vi "test19-AsteriskWildcardStateRegistration.vi"(8 "error in (no error)":errorcluster, 11 "TestCase in":refnum<class "testcase-CSMBroadcast.lvclass">) -> (0 "error out":errorcluster, 3 "TestCase out":refnum<class "testcase-CSMBroadcast.lvclass">)   [LabVIEW 2017, in "testcase-CSMBroadcast.lvclass"]
uses:
  testcase-CSMBroadcast.lvclass
  0c20cacf-7d77-4f8e-aec5-f22e7d09936d.vi
  26de337d-8090-412f-9da5-e117a55d4726.vi
  de10340a-d592-45ad-b055-7fa7b377c551.vi
  e3eae2f8-d8ce-4adb-8167-9a417250fce1.vi
  a4d00e00-a9ed-4631-bf53-269bf71f16fc.vi
  src/user.lib/_NEVSTOP/Communicable State Machine(CSM)/AdvanceAPI/CSM - Revert Arguments-Safe String.vi
  src/user.lib/_NEVSTOP/Communicable State Machine(CSM)/AdvanceAPI/CSM - Make String Arguments Safe.vi
  src/user.lib/_NEVSTOP/Communicable State Machine(CSM)/AdvanceAPI/CSM - Break Down Multiple States String.vi
  src/user.lib/_NEVSTOP/Communicable State Machine(CSM)/AdvanceAPI/CSM - Compact Multiple States.vi
  src/user.lib/_NEVSTOP/Communicable State Machine(CSM)/AdvanceAPI/CSM - Keywords.vi
  src/user.lib/_NEVSTOP/Communicable State Machine(CSM)/_Shared/Trim Single-line Text.vi
  src/user.lib/_NEVSTOP/Communicable State Machine(CSM)/AdvanceAPI/CSM - Set Module Attribute.vi
  src/user.lib/_NEVSTOP/Communicable State Machine(CSM)/AdvanceAPI/CSM - Get Module Attribute.vi
  <vilib>/addons/_JKI Toolkits/VI Tester/TestCase.llb/TestCase.lvclass
  src/user.lib/_NEVSTOP/Communicable State Machine(CSM)/Communicable State Machine.lvlib
  CSM/CSM-Testcase.lvlib
  C:/Program Files (x86)/National Instruments/LabVIEW 2017/vi.lib/addons/_JKI Toolkits/VI Tester/TestCase.llb/TestCase.lvclass
panel:
  out "Execution Times":i32
  out "State History":string
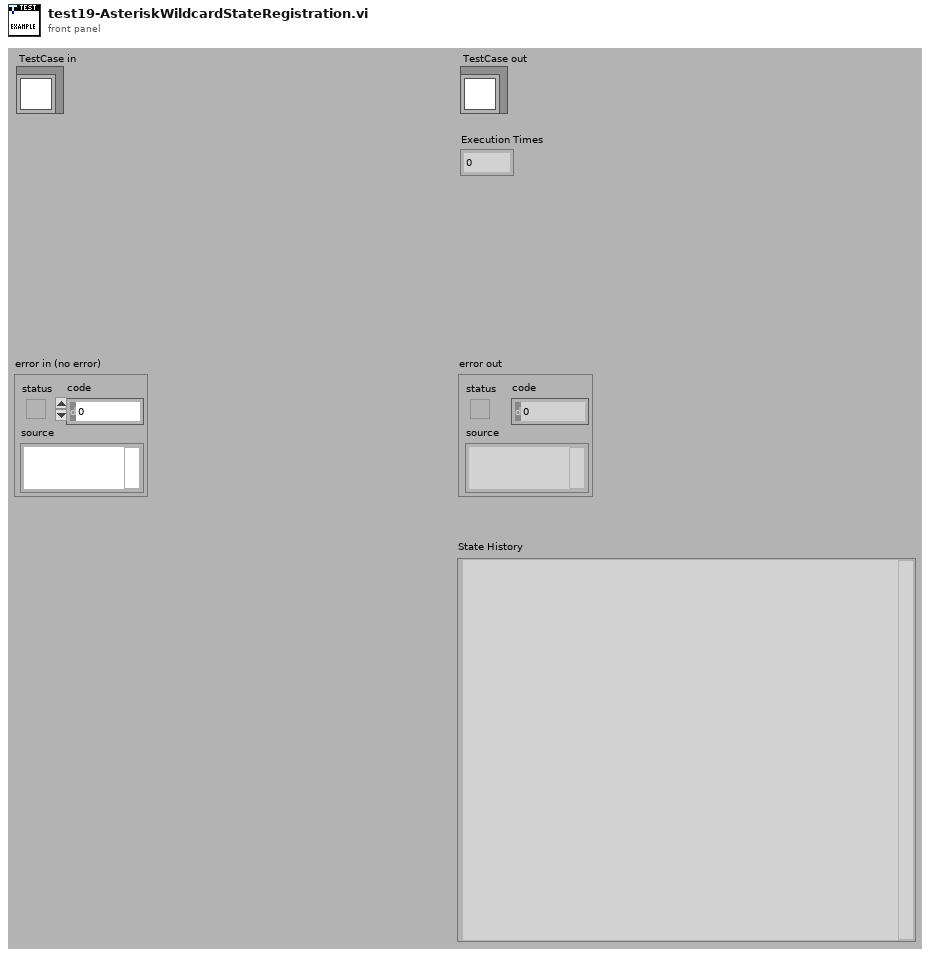
[diagram p1: front panel]
types:
  T1 = enum32{"Invalid", "Standard", "Closed", "Hidden", "Minimized", "Maximized"}
  T2 = enum32{"invalid app kind", "Development System", "Run Time System", "Student Edition", "Embedded LabVIEW", "Evaluation", "Custom"}
  T3 = typedef "Communicable State Machine.lvlib/_CSM_Response Source Message.ctl" = cluster{"‘State":string, "’Arguments":string, "’Error":errorcluster}
  T4 = cluster{"Current VI Reference":refnum<vi>, "Close Panel on Exit?":bool}
  T5 = cluster{"Core":cluster{"Current VI Reference":refnum<vi>, "Close Panel on Exit?":bool}, "Your Boolean data":bool, "Your string data":string, "TestData":i32}
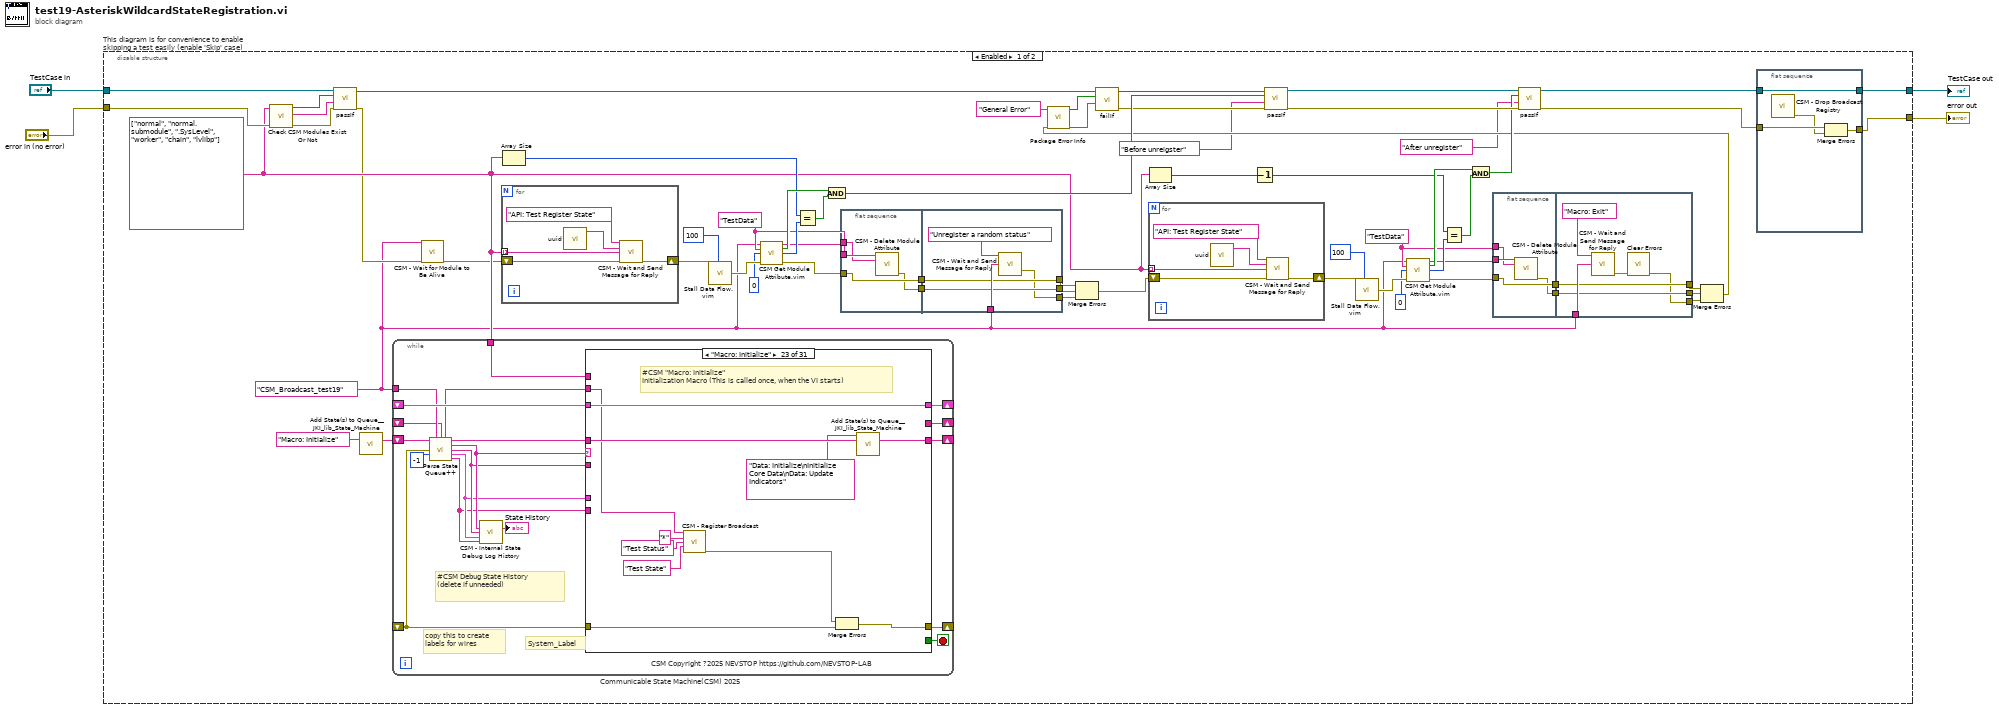
[diagram p0: block diagram]
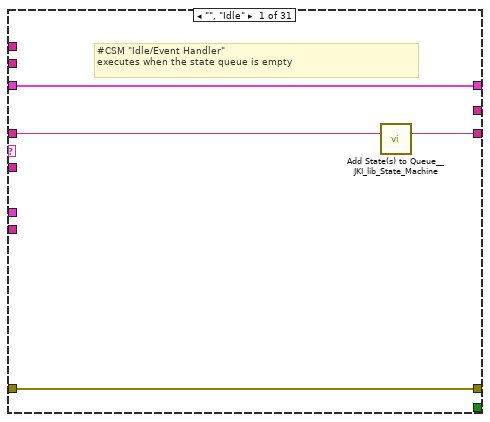
[diagram p2: hidden frame]
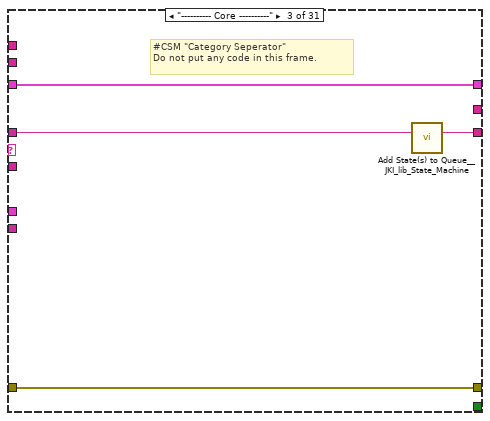
[diagram p4: hidden frame]
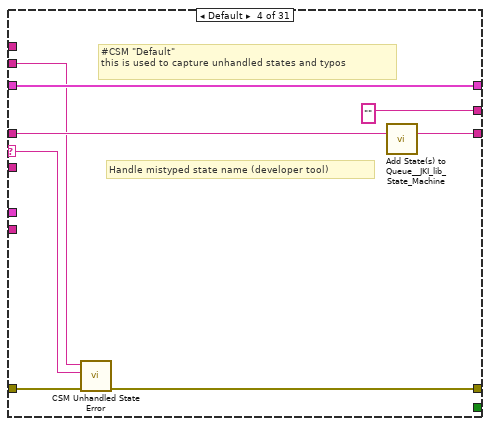
[diagram p5: hidden frame]
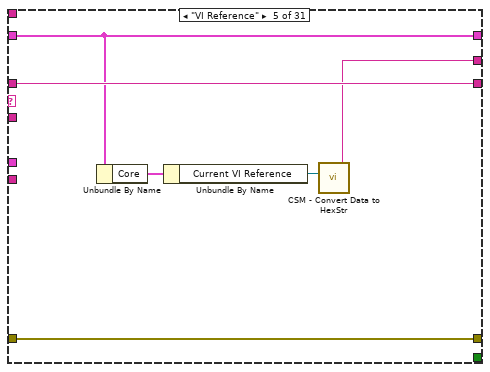
[diagram p6: hidden frame]
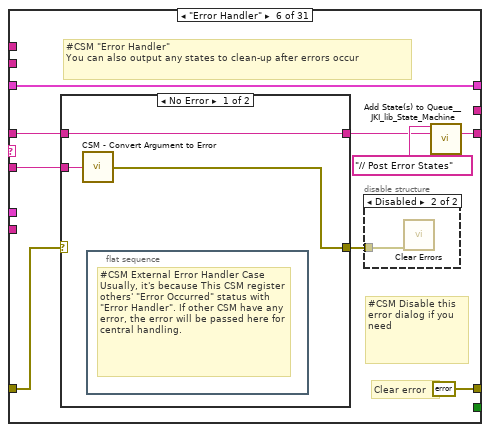
[diagram p7: hidden frame]
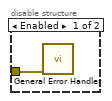
[diagram p8: hidden frame]
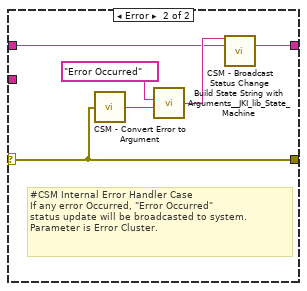
[diagram p9: hidden frame]
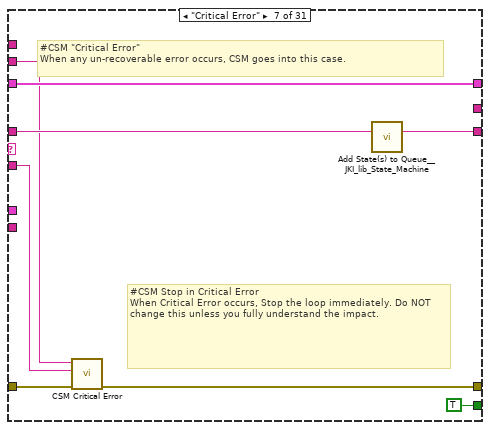
[diagram p10: hidden frame]
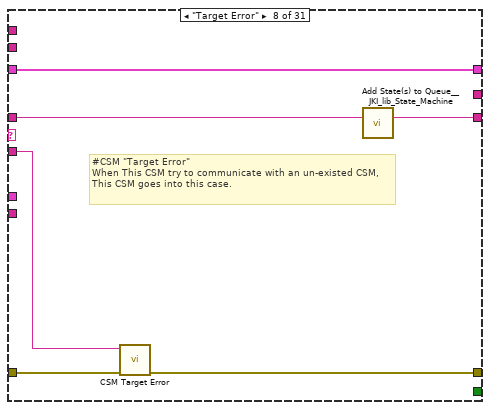
[diagram p11: hidden frame]
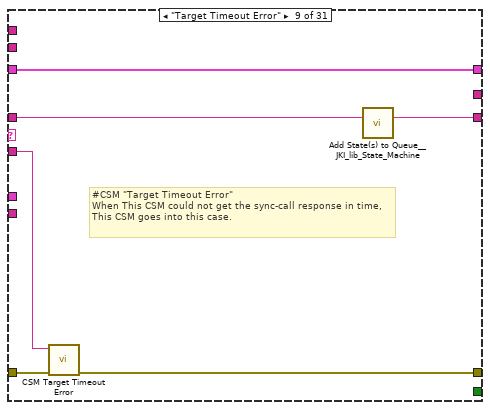
[diagram p12: hidden frame]
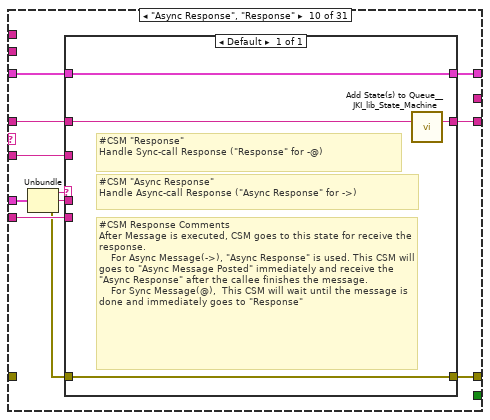
[diagram p13: hidden frame]
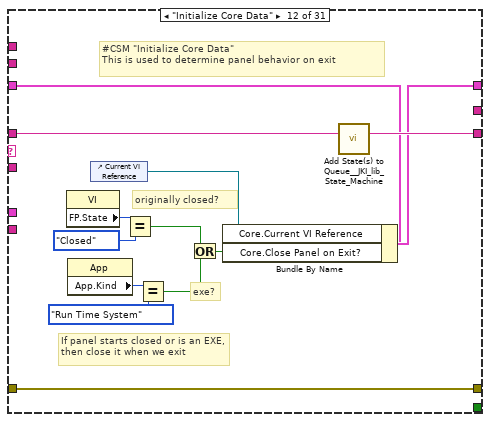
[diagram p15: hidden frame]
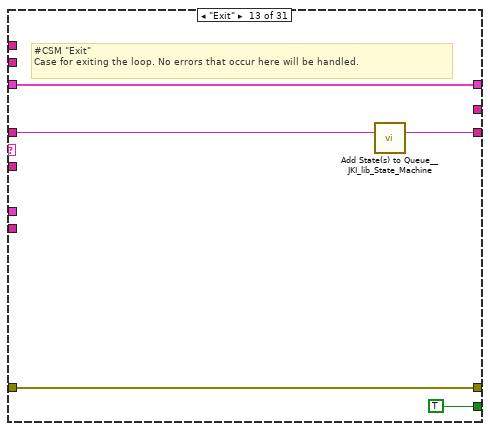
[diagram p16: hidden frame]
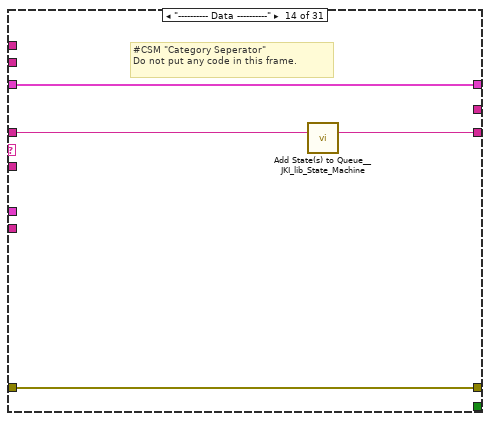
[diagram p17: hidden frame]
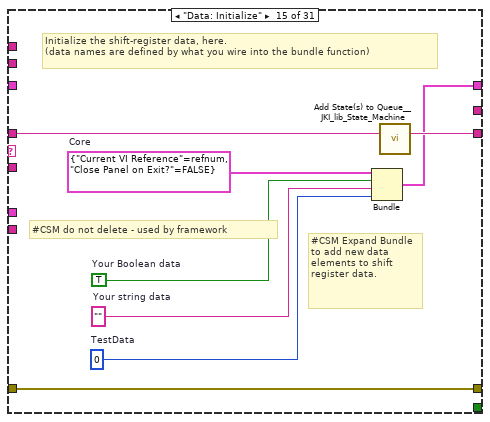
[diagram p18: hidden frame]
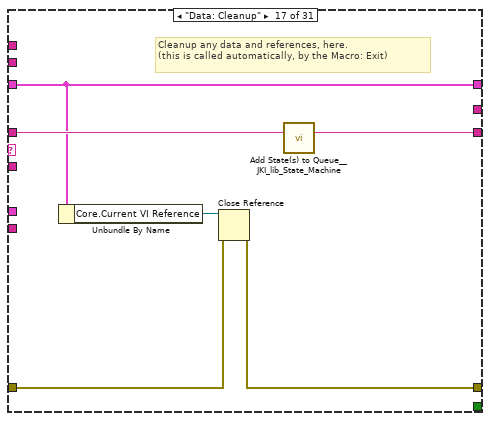
[diagram p20: hidden frame]
diagram:
  n1 = disable-structure "This diagram is for convenience to enable skipping a test easily (enable 'Skip' case)" shown="Enabled" {
    disable-tunnel: "TestCase in" -> [w23 w419]
    disable-tunnel: [w18 w417] -> w1
    disable-tunnel: [w17 w418] -> w3
    disable-tunnel: "error in (no error)" -> [w22 w416]
    frame Enabled {
      w32 = "TestData" ("Attribute")
      w54 = "TestData" ("Attribute")
      w5 = "CSM_Broadcast_test19" ("Name (\"\" to Use UUID)")
      w21 = string[] ["normal", "normal.submodule", ".SysLevel", "worker", "chain", "lvlibp"]
      n2 = call "Check CSM Modules Exist Or Not.vi"("error in"=w22, "CSM names in"=w21) -> ("error out"=w24:errorcluster, "Debug string"=w25:string, "All Modules Exist?"=w26:bool)  [unwired: 7 in]
      n3 = call-dynamic "passIf.vi"("error in (no error)"=w24, "message (\"\")"=w25, "pass"=w26, "TestCase in"=w23) -> ("error out"=w6:errorcluster, "TestCase out"=w15:refnum<class "testcase-CSMBroadcast.lvclass">)  [unwired: 6 in]
      n4 = call <vilib>:"Add State(s) to Queue__JKI_lib_State_Machine.vi"("State(s) in (\"\")"="Macro: Initialize" ("Init State(\"Macro: Initialize\")")) -> ("States Out"=w65:string)  [unwired: 14 in]
      n5 = while "Communicable State Machine(CSM) 2025" {
        shift-right: [w108] -> _
        shift-left: _ -> [w107]
        shift-right: [w111] -> _
        shift-left: _ -> [w106]
        shift-right: [w110] -> _
        shift-left: w65 -> [w112]
        tunnel: w5 -> [w104]
        shift-right: [w105] -> _
        shift-left: _ -> [w98]
        tunnel: w21 -> [w95]
        stop <- w109 stop-if-true
        # "#CSM Debug State History\n(delete if unneeded)"
        # "copy this to create labels for wires"
        # "System_Label"
        # "CSM Copyright ?2025 NEVSTOP https://github.com/NEVSTOP-LAB"
        n6 = call "Parse State Queue++.vi"("State Queue"=w112, "Name (\"\" to Use UUID)"=w104, "Response Arguments"=w98, "Previous Error"=w106, "Dequeue (1 ms)"=-1 ("Timeout")) -> ("Name Used"=w99:string, "Remaining States"=w113:string, "Current State"=w103:string, "Arguments"=w102:string, "Additional Information"=w101:T3, "Source CSM"=w100:string)  [unwired: 5 in]
        n7 = call "CSM - Internal State Debug Log History.vi"("State"=w103, "Arguments (\"\")"=w102, ">> Response Source Message >>"=w101, "Source (\"\")"=w100) -> ("Debug Log"=→"State History":string)  [unwired: 11 in]
        n8 = case shown="\"Macro: Initialize\"" w103 {
          selector: w103 -> [_ _ _ w127 _ _ _ _ _ _ _ _ _ _ _ _ _ _ _ _ _ _ _ _ _ _ _ _ _ _ _]
          tunnel: w113 -> [w114 w119 w124 w131 w137 w143 w164 w170 w176 w184 w195 w209 w214 w218 w226 w228 w235 w239 w243 w249 w264 w333 w344 w357 w359 w363 w368 w375 w379 w390 w410]
          tunnel: w102 -> [_ _ _ _ _ w142 w160 w169 w174 w183 _ _ _ _ _ _ _ _ _ w244 w258 _ _ _ _ _ w366 _ _ _ _]
          tunnel: w107 -> [w115 w118 w121 w129 w136 w146 w165 w171 w177 w186 w194 w202 w212 w215 _ w227 w230 w236 w241 w247 w260 w330 w341 w354 w358 w362 w367 w372 w376 w382 w396]
          tunnel: [w116 w120 w122 w125 w138 errorcluster {"status"=FALSE, "code"=0, "source"=""} ("error out") w161 w167 w173 w189 w196 w206 w211 w216 w223 w229 w231 w237 w240 w245 w261 w331 w335 w346 w360 w364 w369 w373 w377 w384 w398] -> w111
          tunnel: w106 -> [w116 w120 w122 w132 w138 w144 w166 w168 w175 _ w196 w206 w211 w216 w223 w229 w232 w237 w240 w246 w262 w331 w342 w355 w360 w364 w369 w373 w377 w388 w408]
          tunnel: [w117 w119 w123 w130 w137 w139 w163 w172 w178 w185 w195 w208 w213 w217 w225 w228 w234 w238 w242 w248 w263 w332 w343 w356 w359 w363 w368 w374 w378 w389 w409] -> w110
          tunnel: [_ _ _ _ _ _ TRUE _ _ _ _ _ TRUE _ _ _ _ _ _ _ _ _ _ _ _ _ _ _ _ _ _] -> w109
          tunnel: [w115 w118 w121 w129 w136 w146 w165 w171 w177 w187 w194 w207 w212 w215 w224 w227 w230 w236 w241 w247 w260 w330 w341 w354 w358 w362 w367 w372 w376 w386 w394] -> w108
          tunnel: w100 -> [_ _ _ _ _ _ _ _ _ w181 _ _ _ _ _ _ _ _ _ _ _ _ _ _ _ _ _ _ _ _ _]
          tunnel: w101 -> [_ _ _ _ _ _ _ _ _ w188 _ _ _ _ _ _ _ _ _ _ _ _ _ _ _ _ _ _ _ _ _]
          tunnel: [_ _ _ "" w133 _ _ _ _ _ _ _ _ _ _ _ _ _ _ _ _ _ _ _ _ "API1 Response" w365 _ _ _ _] -> w105
          tunnel: w99 -> [_ _ _ w126 _ _ w159 _ _ _ _ _ _ _ _ _ _ _ _ _ _ _ w336 w348 _ _ _ _ _ w385 w405]
          tunnel: w95 -> [_ _ _ _ _ _ _ _ _ _ _ _ _ _ _ _ _ _ _ _ _ _ _ _ _ _ _ _ _ _ w401]
          frame "", "Idle" {
            # "#CSM \"Idle/Event Handler\"\nexecutes when the state queue is empty"
            n9 = call <vilib>:"Add State(s) to Queue__JKI_lib_State_Machine.vi"("State(s) in (\"\")"=w114) -> ("States Out"=w117:string)  [unwired: 14 in]
          }
          frame "CSM Documentation" {
            # "#CSM README FIRST\n\nCommunicable State Machine(CSM) is a LabVIEW application framework that builds upon JKI State Machine(JKISM). It follows the pattern of JKISM and extends the keywords to describe message communication between modules, including concepts such as Sync-Message, Async-Message, Subscription/Unsubscription of status - essential elements for creating reusable code modules. For more information, please visit the CSM wiki: https://nevstop-lab.github.io/CSM-Wiki/\n\nFor instructions on JKI State Machine, visit: http://jki.net/state-machine/\nFor information about CSM, visit: https://github.com/NEVSTOP-LAB"
            # "#CSM \"Documentation\"\nCase for holding CSM Documenation"
          }
          frame "---------- Core ----------" {
            # "#CSM \"Category Seperator\"\nDo not put any code in this frame."
            n10 = call <vilib>:"Add State(s) to Queue__JKI_lib_State_Machine.vi"("State(s) in (\"\")"=w124) -> ("States Out"=w123:string)  [unwired: 14 in]
          }
          frame Default {
            # "#CSM \"Default\"\nthis is used to capture unhandled states and typos"
            # "Handle mistyped state name (developer tool)"
            n11 = call "CSM Unhandled State Error.vi"("error in (no error)"=w132, "Undefined State"=w127, "CSM Name"=w126) -> ("error out"=w125:errorcluster)  [unwired: 8 in]
            n12 = call <vilib>:"Add State(s) to Queue__JKI_lib_State_Machine.vi"("State(s) in (\"\")"=w131) -> ("States Out"=w130:string)  [unwired: 14 in]
          }
          frame "VI Reference" {
            n13 = Unbundle By Name(w136) -> ("Core"=w135:T4)
            n14 = Unbundle By Name(w135) -> ("Current VI Reference"=w134:refnum<vi>)
            n15 = call "CSM - Convert Data to HexStr.vi"("Variant"=w134) -> ("HEX String (0-9,A-F)"=w133:string)  [unwired: 8 in]
          }
          frame "Error Handler" {
            # "#CSM Disable this error dialog if you need"
            # "#CSM \"Error Handler\"\nYou can also output any states to clean-up after errors occur"
            # "Clear error"
            n16 = case shown="No Error" w144 {
              selector: w144 -> [_ w153]
              tunnel: [w152 w155] -> w140
              tunnel: w143 -> [w152 w154]
              tunnel: w142 -> [w151 _]
              tunnel: [w150 w153] -> w145
              frame No Error {
                n17 = call "CSM - Convert Argument to Error.vi"("Argument"=w151) -> ("Error"=w150:errorcluster)  [unwired: 4 in]
                n18 = flat-sequence {
                  frame #0 {
                    # "#CSM External Error Handler Case\nUsually, it's because This CSM register others' \"Error Occurred\" status with \"Error Handler\". If other CSM have any error, the error will be passed here for central handling."
                  }
                }
              }
              frame Error {
                # "#CSM Internal Error Handler Case \nIf any error Occurred, \"Error Occurred\" \nstatus update will be broadcasted to system.\nParameter is Error Cluster."
                n19 = call "CSM - Convert Error to Argument.vi"("Error"=w153) -> ("Argument"=w157:string)  [unwired: 4 in]
                n20 = call <vilib>:"Build State String with Arguments__JKI_lib_State_Machine.vi"("Arguments (\"\")"=w157, "State"="Error Occurred" ("Status with Arguments")) -> ("State with Arguments"=w156:string)  [unwired: 4 in]
                n21 = call "CSM - Broadcast Status Change.vi"("Status With Arguments"=w156, "State Queue"=w154) -> ("Remaining States"=w155:string)  [unwired: 13 in]
              }
            }
            n22 = disable-structure shown="Disabled" {
              disable-tunnel: w145 -> [w148 w149]
              frame Enabled {
                n23 = call <vilib>:"General Error Handler.vi"("error in (no error)"=w148) -> ()  [unwired: 10 in, 5 out]
              }
              frame Disabled {
                n24 = call <vilib>:"Clear Errors.vi"("error in (no error)"=w149) -> ()  [unwired: 5 in, 2 out]
              }
            }
            n25 = call <vilib>:"Add State(s) to Queue__JKI_lib_State_Machine.vi"("State(s) in Front (\"\")"="// Post Error States", "State(s) in (\"\")"=w140) -> ("States Out"=w139:string)  [unwired: 13 in]
          }
          frame "Critical Error" {
            # "#CSM Stop in Critical Error\nWhen Critical Error occurs, Stop the loop immediately. Do NOT change this unless you fully understand the impact."
            # "#CSM \"Critical Error\"\nWhen any un-recoverable error occurs, CSM goes into this case."
            n26 = call "CSM Critical Error.vi"("error in (no error)"=w166, "Arugments (As Reason)"=w160, "CSM Name"=w159) -> ("error out"=w161:errorcluster)  [unwired: 8 in]
            n27 = call <vilib>:"Add State(s) to Queue__JKI_lib_State_Machine.vi"("State(s) in (\"\")"=w164) -> ("States Out"=w163:string)  [unwired: 14 in]
          }
          frame "Target Error" {
            # "#CSM \"Target Error\"\nWhen This CSM try to communicate with an un-existed CSM, This CSM goes into this case."
            n28 = call "CSM Target Error.vi"("error in (no error)"=w168, "Arguments (As CSM Name)"=w169) -> ("error out"=w167:errorcluster)  [unwired: 9 in]
            n29 = call <vilib>:"Add State(s) to Queue__JKI_lib_State_Machine.vi"("State(s) in (\"\")"=w170) -> ("States Out"=w172:string)  [unwired: 14 in]
          }
          frame "Target Timeout Error" {
            # "#CSM \"Target Timeout Error\"\nWhen This CSM could not get the sync-call response in time, This CSM goes into this case."
            n30 = call "CSM Target Timeout Error.vi"("error in (no error)"=w175, "Arguments (As CSM Name)"=w174) -> ("error out"=w173:errorcluster)  [unwired: 9 in]
            n31 = call <vilib>:"Add State(s) to Queue__JKI_lib_State_Machine.vi"("State(s) in (\"\")"=w176) -> ("States Out"=w178:string)  [unwired: 14 in]
          }
          frame "Async Response", "Response" {
            n32 = Unbundle(w188) -> ("‘State"=w182:string, "’Arguments"=w180:string, "’Error"=w179:errorcluster)
            n33 = case shown="Default" w182 {
              tunnel: [w193] -> w189
              tunnel: w179 -> [w193]
              tunnel: [w192] -> w187
              tunnel: w186 -> [w192]
              tunnel: [w190] -> w185
              tunnel: w184 -> [w191]
              tunnel: w183 -> [_]
              tunnel: w181 -> [_]
              tunnel: w180 -> [_]
              frame Default {
                # "#CSM Response Comments\nAfter Message is executed, CSM goes to this state for receive the response.\n    For Async Message(->), \"Async Response\" is used. This CSM will goes to \"Async Message Posted\" immediately and receive the \"Async Response\" after the callee finishes the message.\n    For Sync Message(@),  This CSM will wait until the message is done and immediately goes to \"Response\""
                # "#CSM \"Async Response\"\nHandle Async-call Response (\"Async Response\" for ->)"
                # "#CSM \"Response\"\nHandle Sync-call Response (\"Response\" for -@)"
                n34 = call <vilib>:"Add State(s) to Queue__JKI_lib_State_Machine.vi"("State(s) in (\"\")"=w191) -> ("States Out"=w190:string)  [unwired: 14 in]
              }
            }
          }
          frame "Async Message Posted" {
            # "#CSM \"Async Message Posted\"\nAfter Async Message is posted (-> or ->| ), CSM goes to this state for post-action.\nYou can use Argument - State to tell which Async Message is called."
          }
          frame "Initialize Core Data" {
            # "#CSM \"Initialize Core Data\"\nThis is used to determine panel behavior on exit"
            # "originally closed?"
            # "exe?"
            # "If panel starts closed or is an EXE, then close it when we exit"
            n35 = property class="VI"() -> ("FP.State"=w199:T1)  [unwired: 2 in, 2 out]
            n36 = property class="App"() -> ("App.Kind"=w205:T2)  [unwired: 2 in, 2 out]
            n37 = control-ref of="Current VI Reference"() -> (w200:refnum<vi>)
            n38 = Equal?(x=w199, y=T1."Closed" ("Front Panel Window:State")) -> (x = y?=w197:bool)
            n39 = Equal?(x=w205, y=T2."Run Time System" ("Application:Kind")) -> (x = y?=w203:bool)
            n40 = Or(x=w197, y=w203) -> (x .or. y?=w201:bool)
            n41 = Bundle By Name(cluster=w202, "Core.Current VI Reference"=w200, "Core.Close Panel on Exit?"=w201) -> (w207:T5)
            n42 = call <vilib>:"Add State(s) to Queue__JKI_lib_State_Machine.vi"("State(s) in (\"\")"=w209) -> ("States Out"=w208:string)  [unwired: 14 in]
          }
          frame "Exit" {
            # "#CSM \"Exit\"\nCase for exiting the loop. No errors that occur here will be handled."
            n43 = call <vilib>:"Add State(s) to Queue__JKI_lib_State_Machine.vi"("State(s) in (\"\")"=w214) -> ("States Out"=w213:string)  [unwired: 14 in]
          }
          frame "---------- Data ----------" {
            # "#CSM \"Category Seperator\"\nDo not put any code in this frame."
            n44 = call <vilib>:"Add State(s) to Queue__JKI_lib_State_Machine.vi"("State(s) in (\"\")"=w218) -> ("States Out"=w217:string)  [unwired: 14 in]
          }
          frame "Data: Initialize" {
            w219 = 0  # TestData
            w220 = T4 {"Current VI Reference"=refnum, "Close Panel on Exit?"=FALSE}  # Core
            w222 = TRUE  # Your Boolean data
            w221 = ""  # Your string data
            # "#CSM do not delete - used by framework"
            # "#CSM Expand Bundle to add new data elements to shift register data."
            # "Initialize the shift-register data, here.\n(data names are defined by what you wire into the bundle function)"
            n45 = Bundle("Core"=w220, "Your Boolean data"=w222, "Your string data"=w221, "TestData"=w219) -> (w224:T5)  [unwired: 1 in]
            n46 = call <vilib>:"Add State(s) to Queue__JKI_lib_State_Machine.vi"("State(s) in (\"\")"=w226) -> ("States Out"=w225:string)  [unwired: 14 in]
          }
          frame "Data: Update Indicators" {
          }
          frame "Data: Cleanup" {
            # "Cleanup any data and references, here.\n(this is called automatically, by the Macro: Exit)"
            n47 = Unbundle By Name(w230) -> ("Core.Current VI Reference"=w233:refnum<vi>)
            n48 = Close Reference(reference=w233, error in (no error)=w232) -> (error out=w231:errorcluster)
            n49 = call <vilib>:"Add State(s) to Queue__JKI_lib_State_Machine.vi"("State(s) in (\"\")"=w235) -> ("States Out"=w234:string)  [unwired: 14 in]
          }
          frame "---------- UI ----------" {
            # "#CSM \"Category Seperator\"\nDo not put any code in this frame."
            n50 = call <vilib>:"Add State(s) to Queue__JKI_lib_State_Machine.vi"("State(s) in (\"\")"=w239) -> ("States Out"=w238:string)  [unwired: 14 in]
          }
          frame "UI: Initialize" {
            # "#CSM \"UI: Initialize\"\nInitialize the User Interface, here.\n(this is called automatically, by the Macro: Init)"
            n51 = call <vilib>:"Add State(s) to Queue__JKI_lib_State_Machine.vi"("State(s) in (\"\")"=w243) -> ("States Out"=w242:string)  [unwired: 14 in]
          }
          frame "UI: Cursor Set" {
            # "#CSM \"UI: Cursor Set\"\nSet and Unset Cursor Busy.\n(Usage: \"UI: Cursor Set >> Busy|Idle\")"
            # "Argument"
            n52 = disable-structure shown="TARGET_TYPE!=Windows" {
              disable-tunnel: w246 -> [w252 w257]
              disable-tunnel: [w251 w257] -> w245
              disable-tunnel: w244 -> [w250 _]
              frame condition #0 (active) {
                n53 = case shown="\"Idle\", Default" w250 {
                  tunnel: w252 -> [w254 w256]
                  tunnel: [w253 w255] -> w251
                  frame "Idle", Default {
                    n54 = call <vilib>:"Unset Busy.vi"("error in (no error)"=w254) -> ("error out"=w253:errorcluster)  [unwired: 10 in]
                  }
                  frame "Busy" {
                    n55 = call <vilib>:"Set Busy.vi"("error in (no error)"=w256) -> ("error out"=w255:errorcluster)  [unwired: 9 in, 1 out]
                  }
                }
              }
              frame condition #1 {
              }
            }
            n56 = call <vilib>:"Add State(s) to Queue__JKI_lib_State_Machine.vi"("State(s) in (\"\")"=w249) -> ("States Out"=w248:string)  [unwired: 14 in]
          }
          frame "UI: Front Panel State" {
            # "#CSM \"UI: Front Panel State\"\nSet Front Panel Open or Closed\n(Usage: \"UI: Front Panel State >> Open|Close\")"
            # "Argument"
            n57 = Unbundle By Name(w260) -> ("Core.Current VI Reference"=w259:refnum<vi>)
            n58 = call <vilib>:"Add State(s) to Queue__JKI_lib_State_Machine.vi"("State(s) in (\"\")"=w264) -> ("States Out"=w263:string)  [unwired: 14 in]
            n59 = case shown="\"Close\", \"Closed\"" w258 {
              tunnel: w262 -> [w270 w285 w296 w309 w322]
              tunnel: [w272 w286 w298 w311 w324] -> w261
              tunnel: w259 -> [w271 w283 w297 w310 w323]
              frame "Open", "Standard", Default {
                w265 = T1."Standard" ("State")
                n60 = property class="VI"(reference=w271, error in=w270) -> (reference out=w268:refnum<vi>, error out=w269:errorcluster, "FP.State"=w267:T1)
                n61 = Not Equal?(x=w267, y=w265) -> (x != y?=w266:bool)
                n62 = case shown="True" w266 {
                  tunnel: [w276 w278] -> w272
                  tunnel: w269 -> [w275 w278]
                  tunnel: w268 -> [w274 _]
                  tunnel: w265 -> [w273 _]
                  frame True {
                    n63 = invoke class="VI" method="FP.Open"(reference=w274, error in=w275, "Activate"=TRUE, "State"=w273) -> (error out=w276:errorcluster)  [unwired: 1 in, 4 out]
                  }
                  frame False {
                  }
                }
              }
              frame "Close", "Closed" {
                n64 = property class="VI"(reference=w283, error in=w285) -> (reference out=w282:refnum<vi>, error out=w284:errorcluster, "FP.State"=w280:T1)
                n65 = Not Equal?(x=w280, y=T1."Closed" ("Front Panel Window:State")) -> (x != y?=w279:bool)
                n66 = case shown="False" w279 {
                  tunnel: [w287 w290] -> w286
                  tunnel: w284 -> [w287 w289]
                  tunnel: w282 -> [_ w288]
                  frame False {
                  }
                  frame True {
                    n67 = invoke class="VI" method="FP.Close"(reference=w288, error in=w289) -> (error out=w290:errorcluster)  [unwired: 1 in, 2 out]
                  }
                }
              }
              frame "Hidden", "Hide" {
                w291 = T1."Hidden" ("State")
                n68 = property class="VI"(reference=w297, error in=w296) -> (reference out=w294:refnum<vi>, error out=w295:errorcluster, "FP.State"=w293:T1)
                n69 = Not Equal?(x=w293, y=w291) -> (x != y?=w292:bool)
                n70 = case shown="True" w292 {
                  tunnel: [w302 w303] -> w298
                  tunnel: w295 -> [w301 w303]
                  tunnel: w294 -> [w300 _]
                  tunnel: w291 -> [w299 _]
                  frame True {
                    n71 = invoke class="VI" method="FP.Open"(reference=w300, error in=w301, "State"=w299) -> (error out=w302:errorcluster)  [unwired: 2 in, 4 out]
                  }
                  frame False {
                  }
                }
              }
              frame "Minimize", "Minimized" {
                w304 = T1."Minimized" ("State")
                n72 = property class="VI"(reference=w310, error in=w309) -> (reference out=w307:refnum<vi>, error out=w308:errorcluster, "FP.State"=w306:T1)
                n73 = Not Equal?(x=w306, y=w304) -> (x != y?=w305:bool)
                n74 = case shown="True" w305 {
                  tunnel: [w315 w316] -> w311
                  tunnel: w308 -> [w314 w316]
                  tunnel: w307 -> [w313 _]
                  tunnel: w304 -> [w312 _]
                  frame True {
                    n75 = invoke class="VI" method="FP.Open"(reference=w313, error in=w314, "State"=w312) -> (error out=w315:errorcluster)  [unwired: 2 in, 4 out]
                  }
                  frame False {
                  }
                }
              }
              frame "Maximize", "Maximized" {
                w317 = T1."Maximized" ("State")
                n76 = property class="VI"(reference=w323, error in=w322) -> (reference out=w320:refnum<vi>, error out=w321:errorcluster, "FP.State"=w319:T1)
                n77 = Not Equal?(x=w319, y=w317) -> (x != y?=w318:bool)
                n78 = case shown="True" w318 {
                  tunnel: [w328 w329] -> w324
                  tunnel: w321 -> [w327 w329]
                  tunnel: w320 -> [w326 _]
                  tunnel: w317 -> [w325 _]
                  frame True {
                    n79 = invoke class="VI" method="FP.Open"(reference=w326, error in=w327, "State"=w325) -> (error out=w328:errorcluster)  [unwired: 2 in, 4 out]
                  }
                  frame False {
                  }
                }
              }
            }
          }
          frame "---------- Macro ----------" {
            # "#CSM \"Category Seperator\"\nDo not put any code in this frame."
            n80 = call <vilib>:"Add State(s) to Queue__JKI_lib_State_Machine.vi"("State(s) in (\"\")"=w333) -> ("States Out"=w332:string)  [unwired: 14 in]
          }
          frame "Macro: Initialize" {
            # "#CSM \"Macro: Initialize\"\nInitialization Macro (This is called once, when the VI starts)"
            n81 = call "CSM - Register Broadcast.vi"("CSM Name(Empty for Broadcast Event)"=w336, "Source CSM Name (* as Default)"="*", "Trigger"="Test Status" ("Status"), "API (If \"\", Same as Trigger)"="Test State" ("Response Message (If \"\", Same as Source Message)")) -> ("error out"=w334:errorcluster)  [unwired: 10 in, 1 out]
            n82 = Merge Errors(w334, w342) -> (w335:errorcluster)
            n83 = call <vilib>:"Add State(s) to Queue__JKI_lib_State_Machine.vi"("State(s) in Front (\"\")"="Data: Initialize\nInitialize Core Data\nData: Update Indicators", "State(s) in (\"\")"=w344) -> ("States Out"=w343:string)  [unwired: 13 in]
          }
          frame "Macro: Exit" {
            # "#CSM \"Macro: Exit\"\nExit Macro (This is called once, when the VI exits)"
            n84 = call "CSM - Unregister Broadcast.vi"("CSM Name(Empty for Broadcast Event)"=w348, "Source CSM Name (* as Default)"="*", "Trigger"="Test Status" ("Status"), "API (\"*\" as Default)"="Test State" ("Response Message (If \"\", Same as Source Message)")) -> ("error out"=w345:errorcluster)  [unwired: 10 in, 1 out]
            n85 = call <vilib>:"Add State(s) to Queue__JKI_lib_State_Machine.vi"("State(s) in Front (\"\")"="//Exit Sub-Modules ", "State(s) at Back (\"\")"="Data: Cleanup\nExit") -> ("States Out"=w352:string)  [unwired: 13 in]
            n86 = Merge Errors(w345, w355) -> (w346:errorcluster)
            n87 = call <vilib>:"Add State(s) to Queue__JKI_lib_State_Machine.vi"("State(s) in Front (\"\")"=w352, "State(s) in (\"\")"=w357) -> ("States Out"=w356:string)  [unwired: 13 in]
          }
          frame "---------- API ----------" {
            # "#CSM \"Category Seperator\"\nDo not put any code in this frame."
          }
          frame "API: API1" {
            # "#CSM API Example\nCopy/Rename this case for your own API"
            # "#CSM Response\nConnect this to return the response of your API"
            # "#CSM >> Msg/Rep's CSM >>\nIf you need to tell who triggered this state , use this string. If it's this case itself, this string is \"\"."
            # "#CSM >> Arguments >>\nDeal with the parameter if any"
          }
          frame "API: API2" {
            # "#CSM API Example\nCopy/Rename this case for your own API"
            # "unpack Hex String  to Variant\nif complex parameter is needed."
            n88 = call "CSM - Convert HexStr to Data.vi"("HEX String"=w366) -> ()  [unwired: 7 in, 2 out]
            n89 = disable-structure shown="Disabled" {
              disable-tunnel: [w370 "API2 Response"] -> w365
              frame Disabled {
                # "pack variant to hexstr \nif complex response is needed."
                # "complex Response"
                n90 = call "CSM - Convert Data to HexStr.vi"() -> ("HEX String (0-9,A-F)"=w370:string)  [unwired: 9 in]
              }
              frame Enabled {
              }
            }
          }
          frame "---------- Action ----------" {
            # "#CSM \"Category Seperator\"\nDo not put any code in this frame."
            n91 = call <vilib>:"Add State(s) to Queue__JKI_lib_State_Machine.vi"("State(s) in (\"\")"=w375) -> ("States Out"=w374:string)  [unwired: 14 in]
          }
          frame "Action: action1" {
            # "#CSM \"Internal State\"\nThis category is used for holding internal states"
            n92 = call <vilib>:"Add State(s) to Queue__JKI_lib_State_Machine.vi"("State(s) in (\"\")"=w379) -> ("States Out"=w378:string)  [unwired: 14 in]
          }
          frame "Test State" {
            n93 = Unbundle By Name(w382) -> ("TestData"=w387:i32)
            n94 = disable-structure shown="Enabled" {
              frame Disabled {
                n95 = feedback #1(0 ("y")) -> (w392:i32)
                n96 = Increment(x=w392) -> (x+1=w391:i32)
                "Execution Times" <- w391
                n97 = feedback-in #1(w391) -> ()
              }
              frame Enabled {
              }
            }
            n98 = Increment(x=w387) -> (x+1=w380:i32)
            n99 = Bundle By Name(cluster=w382, "TestData"=w380) -> (w386:T5)
            n100 = call "CSM Set Module Attribute.vim"("CSM Name"=w385, "Attribute"="TestData", "Value"=w380) -> ("error out"=w383:errorcluster)  [unwired: 9 in, 3 out]
            n101 = call <vilib>:"Add State(s) to Queue__JKI_lib_State_Machine.vi"("State(s) in (\"\")"=w390) -> ("States Out"=w389:string)  [unwired: 14 in]
            n102 = Merge Errors(w388, w383) -> (w384:errorcluster)
          }
          frame "Unregister a random status" {
            n103 = Random Number (0-1)() -> (number: 0 to 1=w403:dbl)
            n104 = Array Size(array=w401) -> (size(s)=w404:i32)
            n105 = Multiply(x=w404, y=w403) -> (x*y=w402:dbl)
            n106 = Bundle By Name(cluster=w396, "TestData"=0) -> (w394:T5)
            n107 = Round Toward -Infinity(1:w402) -> (0:w400:dbl)
            n108 = Index Array(array=w401, index=w400) -> (element=w399:string)
            n109 = call "CSM - Unregister Broadcast.vi"("CSM Name(Empty for Broadcast Event)"=w405, "Source CSM Name (* as Default)"=w399, "Trigger"="Test Status" ("Status"), "API (\"*\" as Default)"="Test State" ("Response Message (If \"\", Same as Source Message)")) -> ("error out"=w397:errorcluster)  [unwired: 10 in, 1 out]
            n110 = Merge Errors(w408, w397) -> (w398:errorcluster)
            n111 = call <vilib>:"Add State(s) to Queue__JKI_lib_State_Machine.vi"("State(s) in (\"\")"=w410) -> ("States Out"=w409:string)  [unwired: 14 in]
          }
        }
      }
      n112 = call "CSM - Wait for Module to Be Alive.vi"("CSM Name"=w5, "error in (no error)"=w6) -> ("error out"=w7:errorcluster)  [unwired: 11 in, 2 out]
      n113 = for {
        tunnel: w21 -> [w413] mode=indexing
        shift-right: [w412] -> w63
        shift-left: w7 -> [w411]
        n114 = call "uuid.vi"() -> ("UUID"=w414:string)  [unwired: 11 in]
        n115 = call "CSM - Wait and Send Message for Reply.vi"("State"="API: Test Register State", "Arguments (\"\")"=w414, "Target Module"=w413, "Error In (No Error)"=w411) -> ("error out"=w412:errorcluster)  [unwired: 8 in, 3 out]
      }
      n116 = Array Size(array=w21) -> (size(s)=w58:i32)
      n117 = call "Stall Data Flow.vim"("value in"=w63, "milliseconds to wait"=u32 100) -> ("value out"=w62:errorcluster)  [unwired: 1 out]
      n118 = call "CSM Get Module Attribute.vim"("CSM Name"=w5, "Attribute"=w54, "Default Value (Empty Variant)"=0 ("x+1"), "Error In"=w62) -> ("CSM Name (Dup)"=w55:string, "Found"=w60:bool, "Value"=w59:i32, "error out"=w53:errorcluster)  [unwired: 7 in, 1 out]
      n119 = Equal?(x=w58, y=w59) -> (x = y?=w57:bool)
      n120 = And(x=w60, y=w57) -> (x .and. y?=w56:bool)
      n121 = flat-sequence {
        tunnel: w55 -> [w89]
        tunnel: w54 -> [w88]
        tunnel: w53 -> [w87]
        tunnel: [w87] -> w52
        tunnel: [w86] -> w51
        tunnel: w5 -> [w93]
        tunnel: w52 -> [w92]
        tunnel: w51 -> [w91]
        tunnel: [w92] -> w50
        tunnel: [w91] -> w49
        tunnel: [w90] -> w48
        frame #0 {
          n122 = call "CSM - Delete Module Attribute.vi"("CSM Name"=w89, "Attribute"=w88) -> ("error out"=w86:errorcluster)  [unwired: 10 in, 3 out]
        }
        frame #1 {
          n123 = call "CSM - Wait and Send Message for Reply.vi"("State"="Unregister a random status", "Target Module"=w93) -> ("error out"=w90:errorcluster)  [unwired: 10 in, 3 out]
        }
      }
      n124 = Merge Errors(w50, w49, w48) -> (w40:errorcluster)
      n125 = for {
        tunnel: w21 -> [w83] mode=indexing
        shift-right: [w82] -> w46
        shift-left: w40 -> [w81]
        n126 = call "uuid.vi"() -> ("UUID"=w84:string)  [unwired: 11 in]
        n127 = call "CSM - Wait and Send Message for Reply.vi"("State"="API: Test Register State", "Arguments (\"\")"=w84, "Target Module"=w83, "Error In (No Error)"=w81) -> ("error out"=w82:errorcluster)  [unwired: 8 in, 3 out]
      }
      n128 = Array Size(array=w21) -> (size(s)=w39:i32)
      n129 = Decrement(x=w39) -> (x-1=w38:i32)
      n130 = call "Stall Data Flow.vim"("value in"=w46, "milliseconds to wait"=u32 100) -> ("value out"=w45:errorcluster)  [unwired: 1 out]
      n131 = call "CSM Get Module Attribute.vim"("CSM Name"=w5, "Attribute"=w32, "Default Value (Empty Variant)"=0 ("x+1"), "Error In"=w45) -> ("CSM Name (Dup)"=w33:string, "Found"=w43:bool, "Value"=w42:i32, "error out"=w31:errorcluster)  [unwired: 7 in, 1 out]
      n132 = Equal?(x=w38, y=w42) -> (x = y?=w41:bool)
      n133 = And(x=w43, y=w41) -> (x .and. y?=w27:bool)
      n134 = flat-sequence {
        tunnel: w33 -> [w74]
        tunnel: w32 -> [w73]
        tunnel: w31 -> [w72]
        tunnel: [w72] -> w35
        tunnel: [w71] -> w34
        tunnel: w5 -> [w79]
        tunnel: w35 -> [w78]
        tunnel: w34 -> [w77]
        tunnel: [w78] -> w30
        tunnel: [w77] -> w29
        tunnel: [w75] -> w28
        frame #0 {
          n135 = call "CSM - Delete Module Attribute.vi"("CSM Name"=w74, "Attribute"=w73) -> ("error out"=w71:errorcluster)  [unwired: 10 in, 3 out]
        }
        frame #1 {
          n136 = call "CSM - Wait and Send Message for Reply.vi"("State"="Macro: Exit", "Target Module"=w79) -> ("error out"=w76:errorcluster)  [unwired: 10 in, 3 out]
          n137 = call <vilib>:"Clear Errors.vi"("error in (no error)"=w76) -> ("error out"=w75:errorcluster)  [unwired: 5 in, 1 out]
        }
      }
      n138 = Merge Errors(w30, w29, w28) -> (w11:errorcluster)
      n139 = call "Package Error Info.vi"("error in"=w11, "String in"="General Error") -> ("packed error info out"=w12:string, "error status"=w16:bool)  [unwired: 8 in]
      n140 = call-dynamic "failIf.vi"("message (\"\")"=w12, "fail"=w16, "TestCase in"=w15) -> ("error out"=w13:errorcluster, "TestCase out"=w14:refnum<class "testcase-CSMBroadcast.lvclass">)  [unwired: 7 in]
      n141 = call-dynamic "passIf.vi"("error in (no error)"=w13, "message (\"\")"="Before unreigster" ("message (\"\")"), "pass"=w56, "TestCase in"=w14) -> ("error out"=w37:errorcluster, "TestCase out"=w36:refnum<class "testcase-CSMBroadcast.lvclass">)  [unwired: 6 in]
      n142 = call-dynamic "passIf.vi"("error in (no error)"=w37, "message (\"\")"="After unregister" ("message (\"\")"), "pass"=w27, "TestCase in"=w36) -> ("error out"=w19:errorcluster, "TestCase out"=w20:refnum<class "testcase-CSMBroadcast.lvclass">)  [unwired: 6 in]
      n143 = flat-sequence {
        tunnel: w19 -> [w70]
        tunnel: [w69] -> w17
        tunnel: w20 -> [w67]
        tunnel: [w67] -> w18
        frame #0 {
          n144 = call "CSM - Drop Broadcast Registry.vi"() -> ("error out"=w68:errorcluster)  [unwired: 15 in]
          n145 = Merge Errors(w70, w68) -> (w69:errorcluster)
        }
      }
    }
    frame Disabled {
      # "skip test result while test is under development"
      n146 = call <vilib>:"skip.vi"("error in (no error)"=w416, "TestCase in"=w419) -> ("error out"=w418:errorcluster, "TestCase out"=w417:refnum<class "testcase-CSMBroadcast.lvclass">)  [unwired: 8 in]
    }
  }
  "error out" <- w3
  "TestCase out" <- w1
